vi "Write _To_TXT_File.vi"(0 "refnum":refnum<file>, 7 "text":string, 11 "error in":errorcluster) -> (4 "refnum out":refnum<file>, 8 "path":path, 15 "error out":errorcluster)   [LabVIEW 2016]
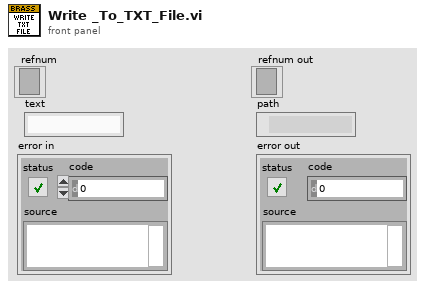
[diagram p1: front panel]
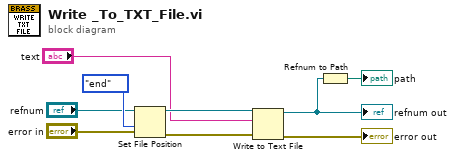
[diagram p0: block diagram]
diagram:
  n1 = Set File Position(refnum="refnum", from (0:start)=enum16{"start", "end", "current"}."end", error in="error in") -> (refnum out=w5:refnum<file>, error out=w6:errorcluster)  [unwired: 1 in]
  n2 = Write to Text File(file (use dialog)=w5, text="text", error in=w6) -> (refnum out=w1:refnum<file>, error out=→"error out":errorcluster)  [unwired: 1 in, 1 out]
  "refnum out" <- w1
  n3 = Refnum to Path(1:w1) -> (0:→"path":path)
